vi "SHGetFolderPath Return Error.vi"(2 "SHGetFolderPath Error Enumeration":T1, 3 "Path":path) -> (0 "error out":errorcluster)   [LabVIEW 2019]
uses:
  SHGetFolderPath Errors.ctl
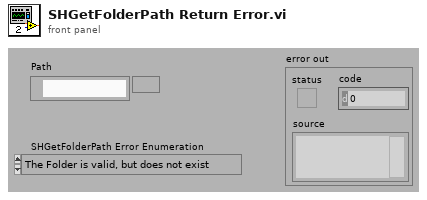
[diagram p1: front panel]
types:
  T1 = typedef "SHGetFolderPath Errors.ctl" = enum16{"The Folder is valid, but does not exist", "An invalid folder ID was specified", "Unrecognized Result from SHFolderPath call"}
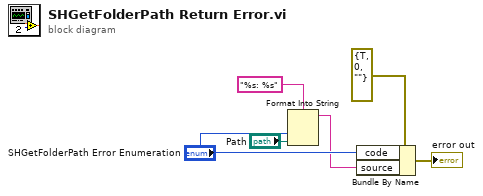
[diagram p0: block diagram]
diagram:
  n1 = Format Into String(format string="%s: %s", "SHGetFolderPath Error Enumeration", "Path") -> (resulting string=w1:string)  [unwired: 2 in, 1 out]
  n2 = Bundle By Name(cluster=errorcluster {"status"=TRUE, "code"=0, "source"=""} ("error out"), "code"="SHGetFolderPath Error Enumeration", "source"=w1) -> (→"error out":errorcluster)
